vi "GetUniqueFiles.vi"(10 "Array in":string[](array[string])) -> (2 "Array out":string[](array[string]))   [LabVIEW 2018]
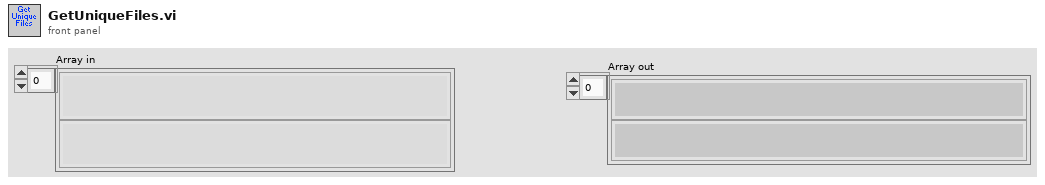
[diagram p1: front panel]
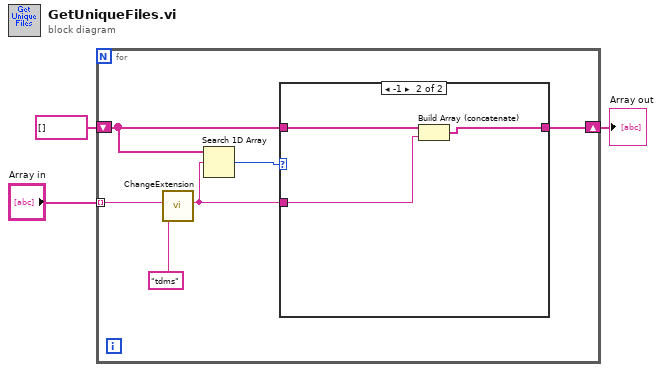
[diagram p0: block diagram]
diagram:
  n1 = for {
    tunnel: "Array in" -> [w5] mode=indexing
    shift-right: [w8] -> w1
    shift-left: string[] [] -> [w7]
    n2 = call "ChangeExtension.vi"("extension"="tdms", "file in"=w5) -> ("file out"=w4:string)  [unwired: 3 in, 4 out]
    n3 = Search 1D Array(1D array=w7, element=w4) -> (index of element=w9:i32)  [unwired: 1 in]
    n4 = case shown="-1" w9 {
      tunnel: [w10 w11] -> w8
      tunnel: w7 -> [w10 w12]
      tunnel: w4 -> [_ w13]
      frame 0, Default {
      }
      frame -1 {
        n5 = Build Array (concatenate)(w12, w13) -> (w11:string[])
      }
    }
  }
  "Array out" <- w1
